vi "Get Signal Data.vi"(8 "error in (no error)":errorcluster, 9 "#s":i32=9800, 10 "channel number":i32=5, 11 "Signal Provider in":refnum<class "Signal Provider.lvclass">) -> (0 "error out":errorcluster, 2 "data":waveform(dbl)(graph), 3 "Signal Provider out":refnum<class "Signal Provider.lvclass">)   [LabVIEW 2019, in "Signal Provider.lvclass"]
uses:
  Signal Provider.lvclass
  Signal Provider.lvclass/Signal Provider.ctl
  <vilib>/measure/NI_MABase.lvlib
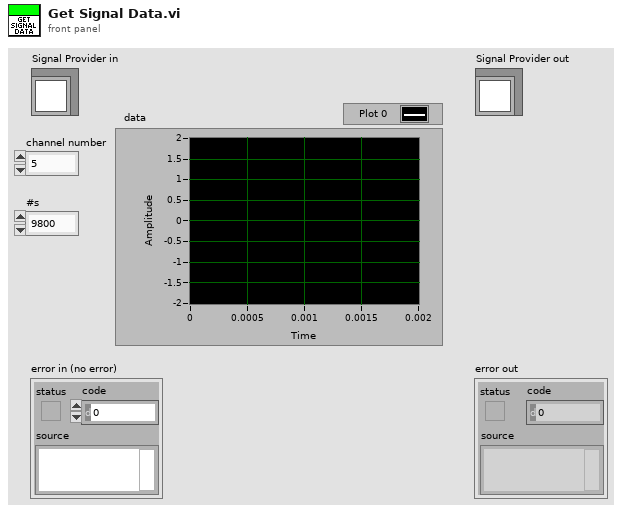
[diagram p1: front panel]
types:
  T1 = enum16{"Sine Wave", "Triangle Wave", "Square Wave", "Sawtooth Wave"}
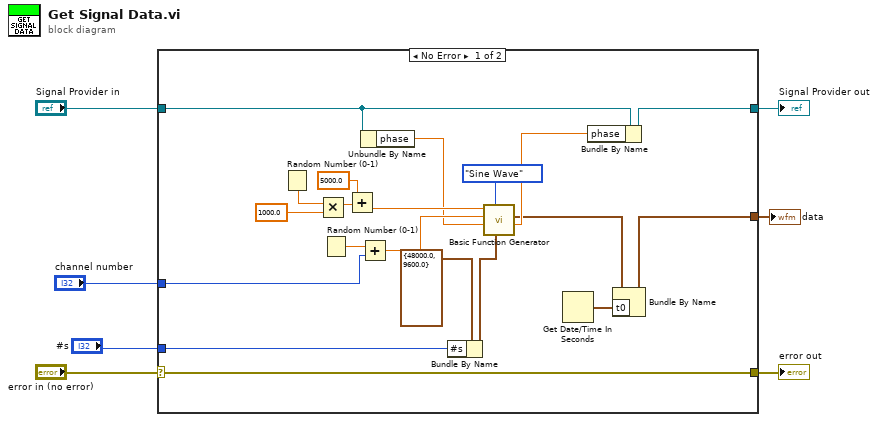
[diagram p0: block diagram]
diagram:
  n1 = case shown="No Error" "error in (no error)" {
    selector: "error in (no error)" -> [w27 w29]
    tunnel: [w27 w29] -> w6
    tunnel: [w19 w28] -> w4
    tunnel: "Signal Provider in" -> [w17 w28]
    tunnel: [w9 _] -> w3
    tunnel: "channel number" -> [w12 _]
    tunnel: "#s" -> [w10 _]
    frame No Error {
      n2 = Random Number (0-1)() -> (number: 0 to 1=w26:dbl)
      n3 = Multiply(x=w26, y=1000.0) -> (x*y=w24:dbl)
      n4 = Random Number (0-1)() -> (number: 0 to 1=w23:dbl)
      n5 = Add(x=5000.0, y=w24) -> (x+y=w21:dbl)
      n6 = Add(x=w23, y=w12) -> (x+y=w22:dbl)
      n7 = Unbundle By Name(w17) -> ("phase"=w16:dbl)
      n8 = Bundle By Name(cluster=cluster{"Fs":dbl, "#s":dbl} {"Fs"=48000.0, "#s"=9600.0} ("sampling info"), "#s"=w10) -> (w11:cluster{"Fs":dbl, "#s":dbl})
      n9 = call <vilib>:"Basic Function Generator.vi"("sampling info"=w11, "signal type"=T1."Sine Wave", "phase"=w16, "amplitude"=w22, "frequency"=w21) -> ("phase out"=w18:dbl, "signal out"=w13:waveform(dbl))  [unwired: 4 in, 1 out]
      n10 = Get Date/Time In Seconds() -> (seconds since 1Jan1904=w8:timestamp)
      n11 = Bundle By Name(cluster=w17, "phase"=w18) -> (w19:refnum<class "Signal Provider.lvclass">)
      n12 = Bundle By Name(cluster=w13, "t0"=w8) -> (w9:waveform(dbl))
    }
    frame Error {
    }
  }
  "error out" <- w6
  "Signal Provider out" <- w4
  "data" <- w3
